vi "SubViWaveToSpreadSheet.vi"(1 "file path (dialog if empty) 3":path, 2 "amplitude":dbl=1.0, 3 "frequency":dbl=50.0 format="%#_13g") -> (0 "dt":dbl)   [LabVIEW 2015]
doc: "Generate a sine wave and write the waveform data into Spreadsheet."
uses:
  <vilib>/Waveform/WDTFileIO.llb/Export Waveform To Spreadsheet File.vi
  <vilib>/measure/NI_MABase.lvlib
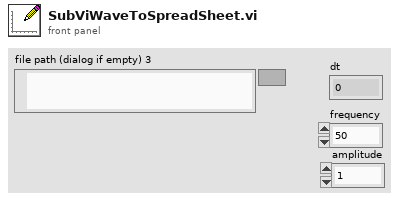
[diagram p1: front panel]
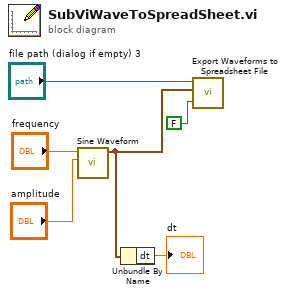
[diagram p0: block diagram]
diagram:
  n1 = call <vilib>:"Sine Waveform.vi"("amplitude"="amplitude", "frequency"="frequency") -> ("signal out"=w1:waveform(dbl))  [unwired: 8 in, 1 out]
  n2 = Unbundle By Name(w1) -> ("dt"=→"dt":dbl)
  n3 = call-poly <vilib>:"Export Waveforms to Spreadsheet File.vi"("header? (write header:T)"=FALSE ("transpose? (F)"), "waveform"=w1, "file path (dialog if empty)"="file path (dialog if empty) 3") -> ()  [unwired: 7 in, 2 out]
